vi "create_full_request_data.vi"(0 "llm_azureopenai_chatmodels in":refnum<class "llm_azureopenai_chatmodels.lvclass">, 5 "Messages":refnum<class "abstract_message_base.lvclass">[](array[class]), 11 "error in (no error)":errorcluster) -> (4 "llm_azureopenai_chatmodels out":refnum<class "llm_azureopenai_chatmodels.lvclass">, 6 "Request Data":string, 15 "error out":errorcluster)   [LabVIEW 2020, in "llm_azureopenai_chatmodels.lvclass"]
uses:
  llm_azureopenai_chatmodels.lvclass
  D:/Personal/LabVIEW LLMs/src/models/abstract_llm_base/abstract_llm_base.lvclass
  abstract_message_base/abstract_message_base.lvclass
  message_text/message_text.lvclass
  llm_openai_chatmodels/llm_openai_chatmodels.lvclass
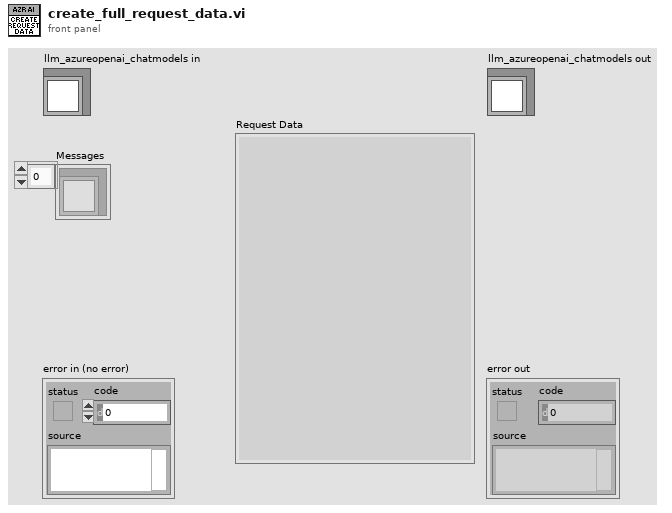
[diagram p1: front panel]
types:
  T1 = cluster{"model":string, "messages":cluster{"role":string, "content":cluster{"type":string, "text":string}[]}[], "temperature":dbl, "max_tokens":u32, "top_p":dbl, "frequency_penalty":dbl, "presence_penalty":dbl}
  T2 = typedef "message_text.lvclass/message.ctl" = cluster{"role":string, "content":string[]}
  T3 = cluster{"role":string, "content":cluster{"type":string, "text":string}[]}
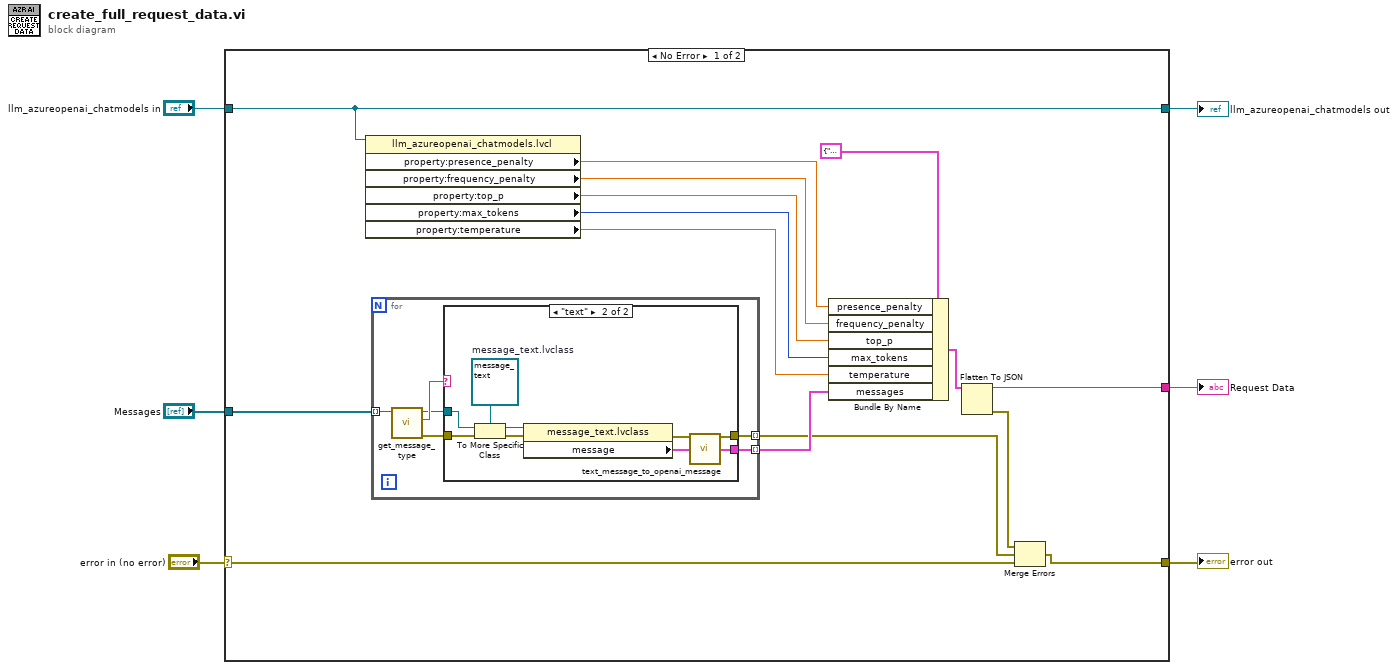
[diagram p0: block diagram]
diagram:
  n1 = case shown="No Error" "error in (no error)" {
    selector: "error in (no error)" -> [w21 w38]
    tunnel: [w16 w38] -> w2
    tunnel: [w12 w37] -> w5
    tunnel: "llm_azureopenai_chatmodels in" -> [w12 w37]
    tunnel: "Messages" -> [w19 _]
    tunnel: [w13 _] -> w1
    frame No Error {
      n2 = property class="llm_azureopenai_chatmodels.lvcl"(reference=w12) -> ("property:presence_penalty"=w11:dbl, "property:frequency_penalty"=w10:dbl, "property:top_p"=w9:dbl, "property:max_tokens"=w8:u32, "property:temperature"=w7:dbl)  [unwired: 1 in, 2 out]
      n3 = for {
        tunnel: w19 -> [w27] mode=indexing
        tunnel: [w23] -> w15 mode=indexing
        tunnel: [w22] -> w18 mode=indexing
        n4 = call-dynamic "get_message_type.vi"("abstract_message_base in"=w27) -> ("error out"=w24:errorcluster, "Type"=w26:string, "abstract_message_base out"=w25:refnum<class "abstract_message_base.lvclass">)  [unwired: 8 in]
        n5 = case shown="\"text\"" w26 {
          tunnel: w25 -> [_ w35]
          tunnel: w24 -> [w28 w36]
          tunnel: [w28 w31] -> w23
          tunnel: [_ w29] -> w22
          frame Default {
          }
          frame "text" {
            w34 = refnum<class "message_text.lvclass"> refnum  # message_text.lvclass
            n6 = To More Specific Class(target class=w34, reference=w35, error in=w36) -> (specific class reference=w33:refnum<class "message_text.lvclass">, error out=w32:errorcluster)
            n7 = property class="message_text.lvclass"(reference=w33, error in=w32) -> (error out=w31:errorcluster, "message"=w30:T2)  [unwired: 1 out]
            n8 = call "text_message_to_openai_message.vi"("message"=w30) -> ("message out"=w29:T3)
          }
        }
      }
      n9 = Bundle By Name(cluster=T1 {"model"="", "messages"=[], "temperature"=1.0, "max_tokens"=256, "top_p"=1.0, "frequency_penalty"=0.0, "presence_penalty"=0.0} ("data"), "presence_penalty"=w11, "frequency_penalty"=w10, "top_p"=w9, "max_tokens"=w8, "temperature"=w7, "messages"=w18) -> (w17:T1)
      n10 = Flatten To JSON(anything=w17) -> (JSON string=w13:string, 11:w14:errorcluster)  [unwired: 2 in]
      n11 = Merge Errors(w14, w15, w21) -> (w16:errorcluster)
    }
    frame Error {
    }
  }
  "error out" <- w2
  "llm_azureopenai_chatmodels out" <- w5
  "Request Data" <- w1
